vi "Configure White Noise.vi"(0 "template configuration":refnum<class "SV Signal.lvclass">, 5 "amplitude PDF":enum16{"Gaussian", "Rectangular", "Triangular"}(ring), 7 "level":dbl=1.0, 9 "seed":i32=-1, 11 "error in (no error)":errorcluster) -> (4 "signal configuration":refnum<class "SV Noise.lvclass">, 15 "error out":errorcluster)   [LabVIEW 2017, in "SV Noise.lvclass"]
doc: "Configures a user-defined test signal. Wire the outputs to SV Signal (waveform) VI to generate the test signal, or wire to SV Signal Property Node to configure additional parameters before wiring to the SV Signal (waveform) VI."
uses:
  <vilib>/addons/_NISVFA/_Generation/Signal Generation/SV Noise/SV Noise.lvclass
  C:/Program Files (x86)/National Instruments/LabVIEW 2017/vi.lib/addons/_NISVFA/_Generation/Signal Generation/SV Signal/SV Signal.lvclass
  <vilib>/addons/_NISVFA/_Generation/Signal Generation/SV Signal/SV Signal.lvclass
  <vilib>/addons/_NISVFA/_Generation/Signal Generation/SV Noise/SV Noise.lvclass/SV Noise.ctl
  <vilib>/addons/_NISVFA/_Generation/Signal Generation/SV Signal/Write Post-Measurement Settling Duration.vi
  <vilib>/addons/_NISVFA/_Generation/Signal Generation/SV Signal/Write Pre-Measurement Settling Duration.vi
  <vilib>/addons/_NISVFA/_Generation/Signal Generation/SV Signal/Write Measurement Duration.vi
  <vilib>/addons/_NISVFA/_Generation/Signal Generation/SV Signal/Write Sample Rate.vi
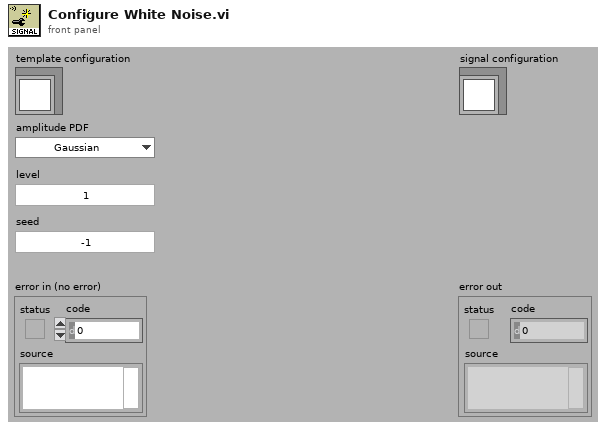
[diagram p1: front panel]
types:
  T1 = enum16{"White noise", "Pink noise", "Periodic random noise"}
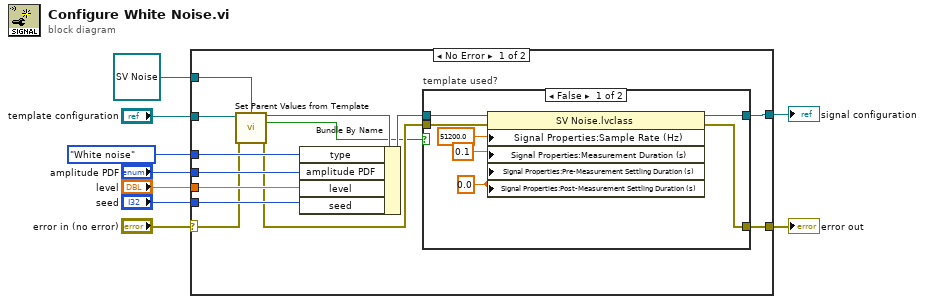
[diagram p0: block diagram]
diagram:
  n1 = case shown="No Error" "error in (no error)" {
    selector: "error in (no error)" -> [w12 w32]
    tunnel: [w16 w32] -> w8
    tunnel: [w17 w33] -> w3
    tunnel: refnum<class "SV Noise.lvclass"> refnum ("BroadbandNoise in") -> [w14 w33]
    tunnel: T1."White noise" ("type") -> [w22 _]
    tunnel: "level" -> [w21 _]
    tunnel: "seed" -> [w20 _]
    tunnel: "amplitude PDF" -> [w19 _]
    tunnel: "template configuration" -> [w15 _]
    frame No Error {
      n2 = call-dynamic "Set Parent Values from Template.vi"("template configuration"=w15, "signal configuration in"=w14, "error in (no error)"=w12) -> ("signal configuration out"=w13:refnum<class "SV Noise.lvclass">, "template used?"=w10:bool, "error out"=w11:errorcluster)  [unwired: 10 in]
      n3 = Bundle By Name(cluster=w13, "type"=w22, "amplitude PDF"=w19, "level"=w21, "seed"=w20) -> (w18:refnum<class "SV Noise.lvclass">)
      n4 = case "template used?" shown="False" w10 {
        tunnel: w18 -> [w28 w31]
        tunnel: [w27 w31] -> w17
        tunnel: [w26 w30] -> w16
        tunnel: w11 -> [w23 w30]
        frame False {
          w29 = 0.0 ("settling time_s")
          n5 = property class="SV Noise.lvclass"(reference=w28, error in=w23, "Signal Properties:Sample Rate (Hz)"=51200.0 ("SampleRate_Hz"), "Signal Properties:Measurement Duration (s)"=0.1 ("integration time_s"), "Signal Properties:Pre-Measurement Settling Duration (s)"=w29, "Signal Properties:Post-Measurement Settling Duration (s)"=w29) -> (reference out=w27:refnum<class "SV Noise.lvclass">, error out=w26:errorcluster)
        }
        frame True {
        }
      }
    }
    frame Error {
    }
  }
  "error out" <- w8
  "signal configuration" <- w3
